vi "DialogCloneMethod.vi"(0 "LibWriter":refnum<class "LibWriter.lvclass">, 1 "VIItemRefIn":refnum<vi>, 5 "error in (no error)":errorcluster) -> (11 "NewVIDescriptionOut":string caption="New VI Description", 13 "OpenAfter":bool, 14 "LibWriter":refnum<class "LibWriter.lvclass">, 15 "VIItemRefOut":refnum<vi>, 16 "NewVIPath":path, 17 "Cancelled":bool, 18 "LibraryOwners":refnum<vi>[](array[refnum]), 19 "error out":errorcluster)   [LabVIEW 2014, in "LibWriter.lvclass"]
uses:
  <resource>/Framework/Providers/Open_GDS/ClassProviders/LibProvider_BaseClassInterface/LibWriter_class/ClassWriter_class/LibWriter.lvclass
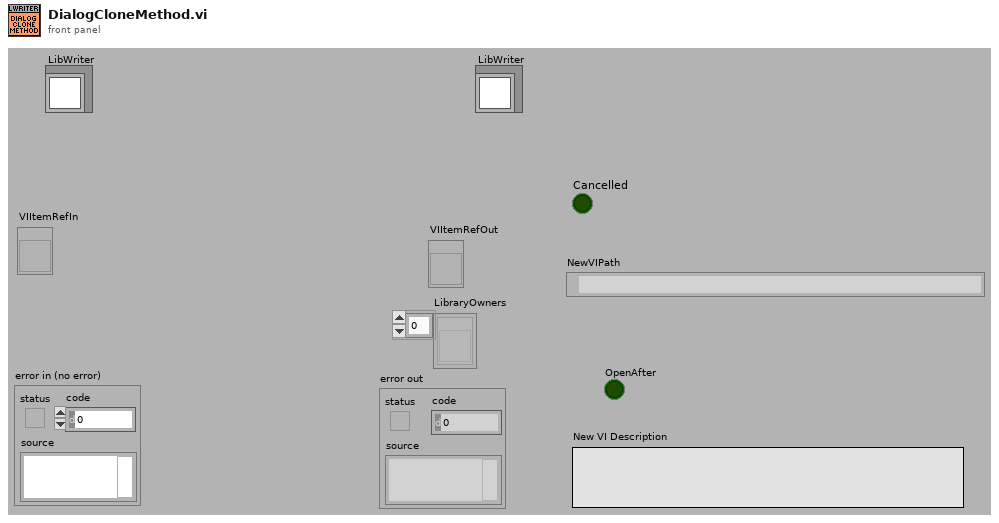
[diagram p1: front panel]
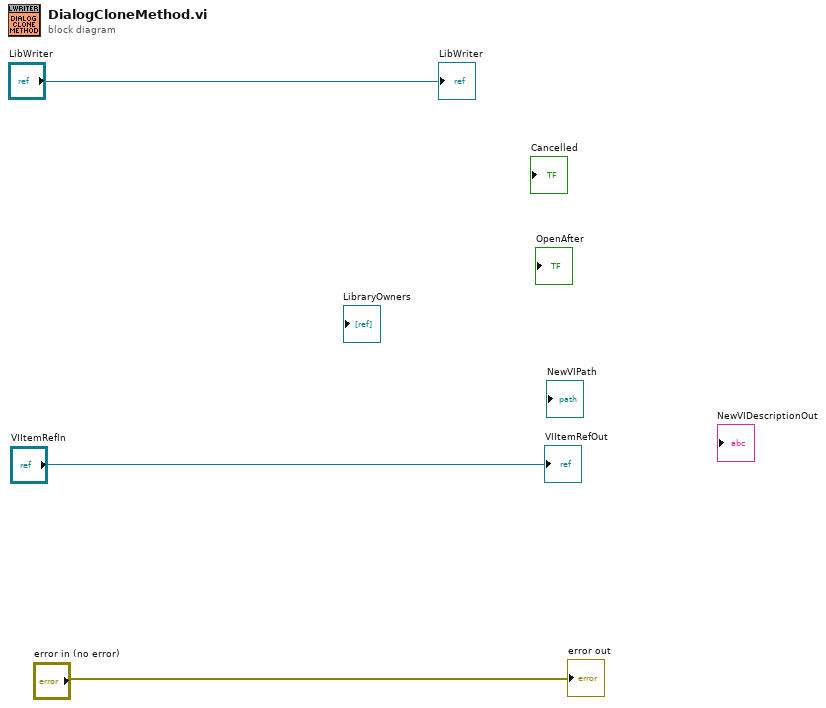
[diagram p0: block diagram]
diagram:
  "VIItemRefOut" <- "VIItemRefIn"
  "error out" <- "error in (no error)"
  "LibWriter" <- "LibWriter"
